vi "Image_set.vi"(8 "error in (no error)":errorcluster, 10 "Image":T1) -> (0 "error out":errorcluster)   [LabVIEW 2009, in "NetworkVarTarget.lvlib"]
uses:
  NetworkVarTarget.lvlib
  <vilib>/vision/Image Controls.llb/IMAQ Image.ctl
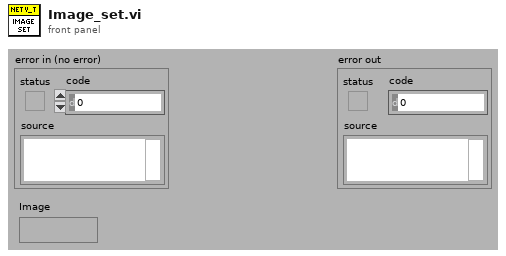
[diagram p1: front panel]
types:
  T1 = typedef "IMAQ Image.ctl" = refnum<image>
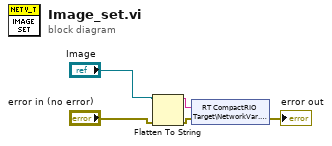
[diagram p0: block diagram]
diagram:
  n1 = Flatten To String(anything="Image", error in (no error)="error in (no error)") -> (data string=w1:string, error out=w2:errorcluster)  [unwired: 2 in, 1 out]
  n2 = shared-variable "RT CompactRIO Target\\NetworkVar.lvlib\\Image"(w1, error in=w2) -> (error out=→"error out":errorcluster)
